vi "认识while循环.vi"() -> ()   [LabVIEW 2018]
panel:
  out "当前总和":i32
  out "当前循环i":i32
  out "字符串":string="while循环先执行后判断，至少执行一次\n目前作用：控制例程停止"
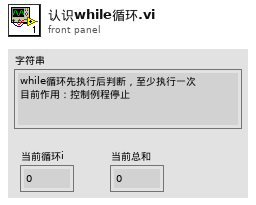
[diagram p1: front panel]
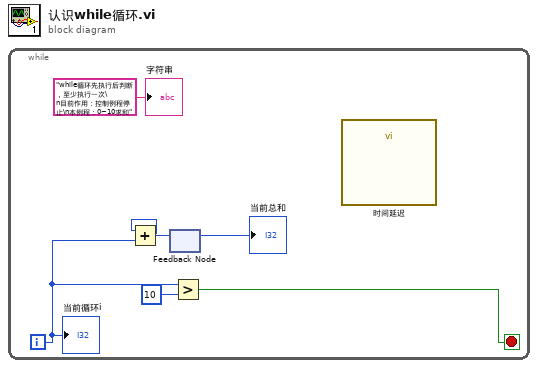
[diagram p0: block diagram]
diagram:
  n1 = while {
    i -> [w3]
    stop <- w1 stop-if-true
    n2 = feedback #1() -> (w4:i32)  [unwired: 1 in]
    "当前总和" <- w4
    n3 = Add(x=w4, y=w3) -> (x+y=w5:i32)
    n4 = feedback-in #1(w5) -> ()
    n5 = Greater?(x=w3, y=10) -> (0:w1:bool)
    n6 = call "时间延迟"() -> ()  [unwired: 11 in, 1 out]
    "字符串" <- "while循环先执行后判断，至少执行一次\n目前作用：控制例程停止\n本例程：0~10求和"
    "当前循环i" <- w3
  }
